vi "Read MFC Data.vi"(8 "error in":errorcluster, 11 "CRDS Data in":refnum<class "CRDS Data.lvclass">) -> (0 "error out":errorcluster, 2 "mfcDataOut":T1(array[cluster]), 3 "CRDS Data out":refnum<class "CRDS Data.lvclass">)   [LabVIEW 2011, in "CRDS Data.lvclass"]
doc: "Retrieve the MFC data from the CRDS Data class and put it in a format that is understandable."
uses:
  CRDS Data.lvclass
  Reusable/DataClass/Alicat/MC/AlicatMCData.lvclass
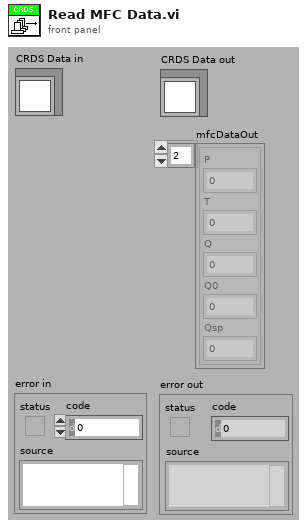
[diagram p1: front panel]
types:
  T1 = cluster{"P":sgl, "T":sgl, "Q":sgl, "Q0":sgl, "Qsp":sgl}[]
  T2 = cluster{"P":sgl, "T":sgl, "Q":sgl, "Q0":sgl, "Qsp":sgl}
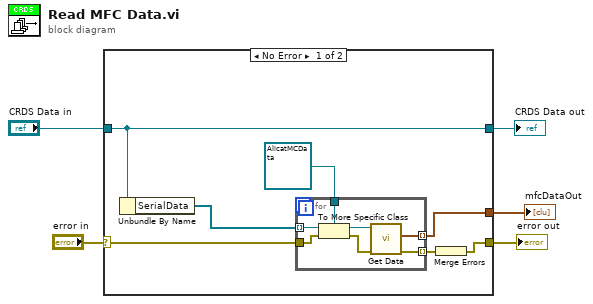
[diagram p0: block diagram]
diagram:
  n1 = case shown="No Error" "error in" {
    selector: "error in" -> [w10 w21]
    tunnel: [w7 w21] -> w4
    tunnel: [w12 w20] -> w2
    tunnel: "CRDS Data in" -> [w12 w20]
    tunnel: [w6 _] -> w1
    frame No Error {
      n2 = Unbundle By Name(w12) -> ("SerialData"=w11:refnum<class "Data.lvclass">[])
      n3 = for {
        tunnel: w11 -> [w19] mode=indexing
        tunnel: w10 -> [w18]
        tunnel: refnum<class "AlicatMCData.lvclass"> refnum ("AlicatMCData.lvclass") -> [w16]
        tunnel: [w14] -> w6 mode=indexing
        tunnel: [w13] -> w8 mode=indexing
        n4 = To More Specific Class(target class=w16, reference=w19, error in=w18) -> (specific class reference=w17:refnum<class "AlicatMCData.lvclass">, error out=w15:errorcluster)
        n5 = call "Get Data.vi"("error in"=w15, "AlicatMData in"=w17) -> ("error out"=w13:errorcluster, "SystemData"=w14:T2)  [unwired: 7 in, 1 out]
      }
      n6 = Merge Errors(w8) -> (w7:errorcluster)
    }
    frame Error {
    }
  }
  "error out" <- w4
  "CRDS Data out" <- w2
  "mfcDataOut" <- w1
